vi "Helium Test - Step 4.vi"(7 "Step":i32, 8 "error in":errorcluster, 9 "Test Results":T9, 10 "Oil In":T1, 11 "Test Configuration":T2) -> (0 "error out":errorcluster, 1 "Test Results Out":T9, 2 "Oil Out":T1, 3 "Test Configuration Out":T2)   [LabVIEW 2015]
uses:
  Controls/Test Results.ctl
  Controls/Step Result.ctl
  Controls/Startup Test.ctl
  Controls/Test Information.ctl
  Controls/Vacuum Test.ctl
  Controls/Test Timing.ctl
  Controls/Vaccum Thresholds.ctl
  Controls/Helium Test.ctl
  Controls/Helium Thresholds.ctl
  Controls/Startup Thresholds.ctl
  CAN Communication/Oil/Typedefs/Session Handle.ctl
  CAN Communication/Oil/Oil.lvclass
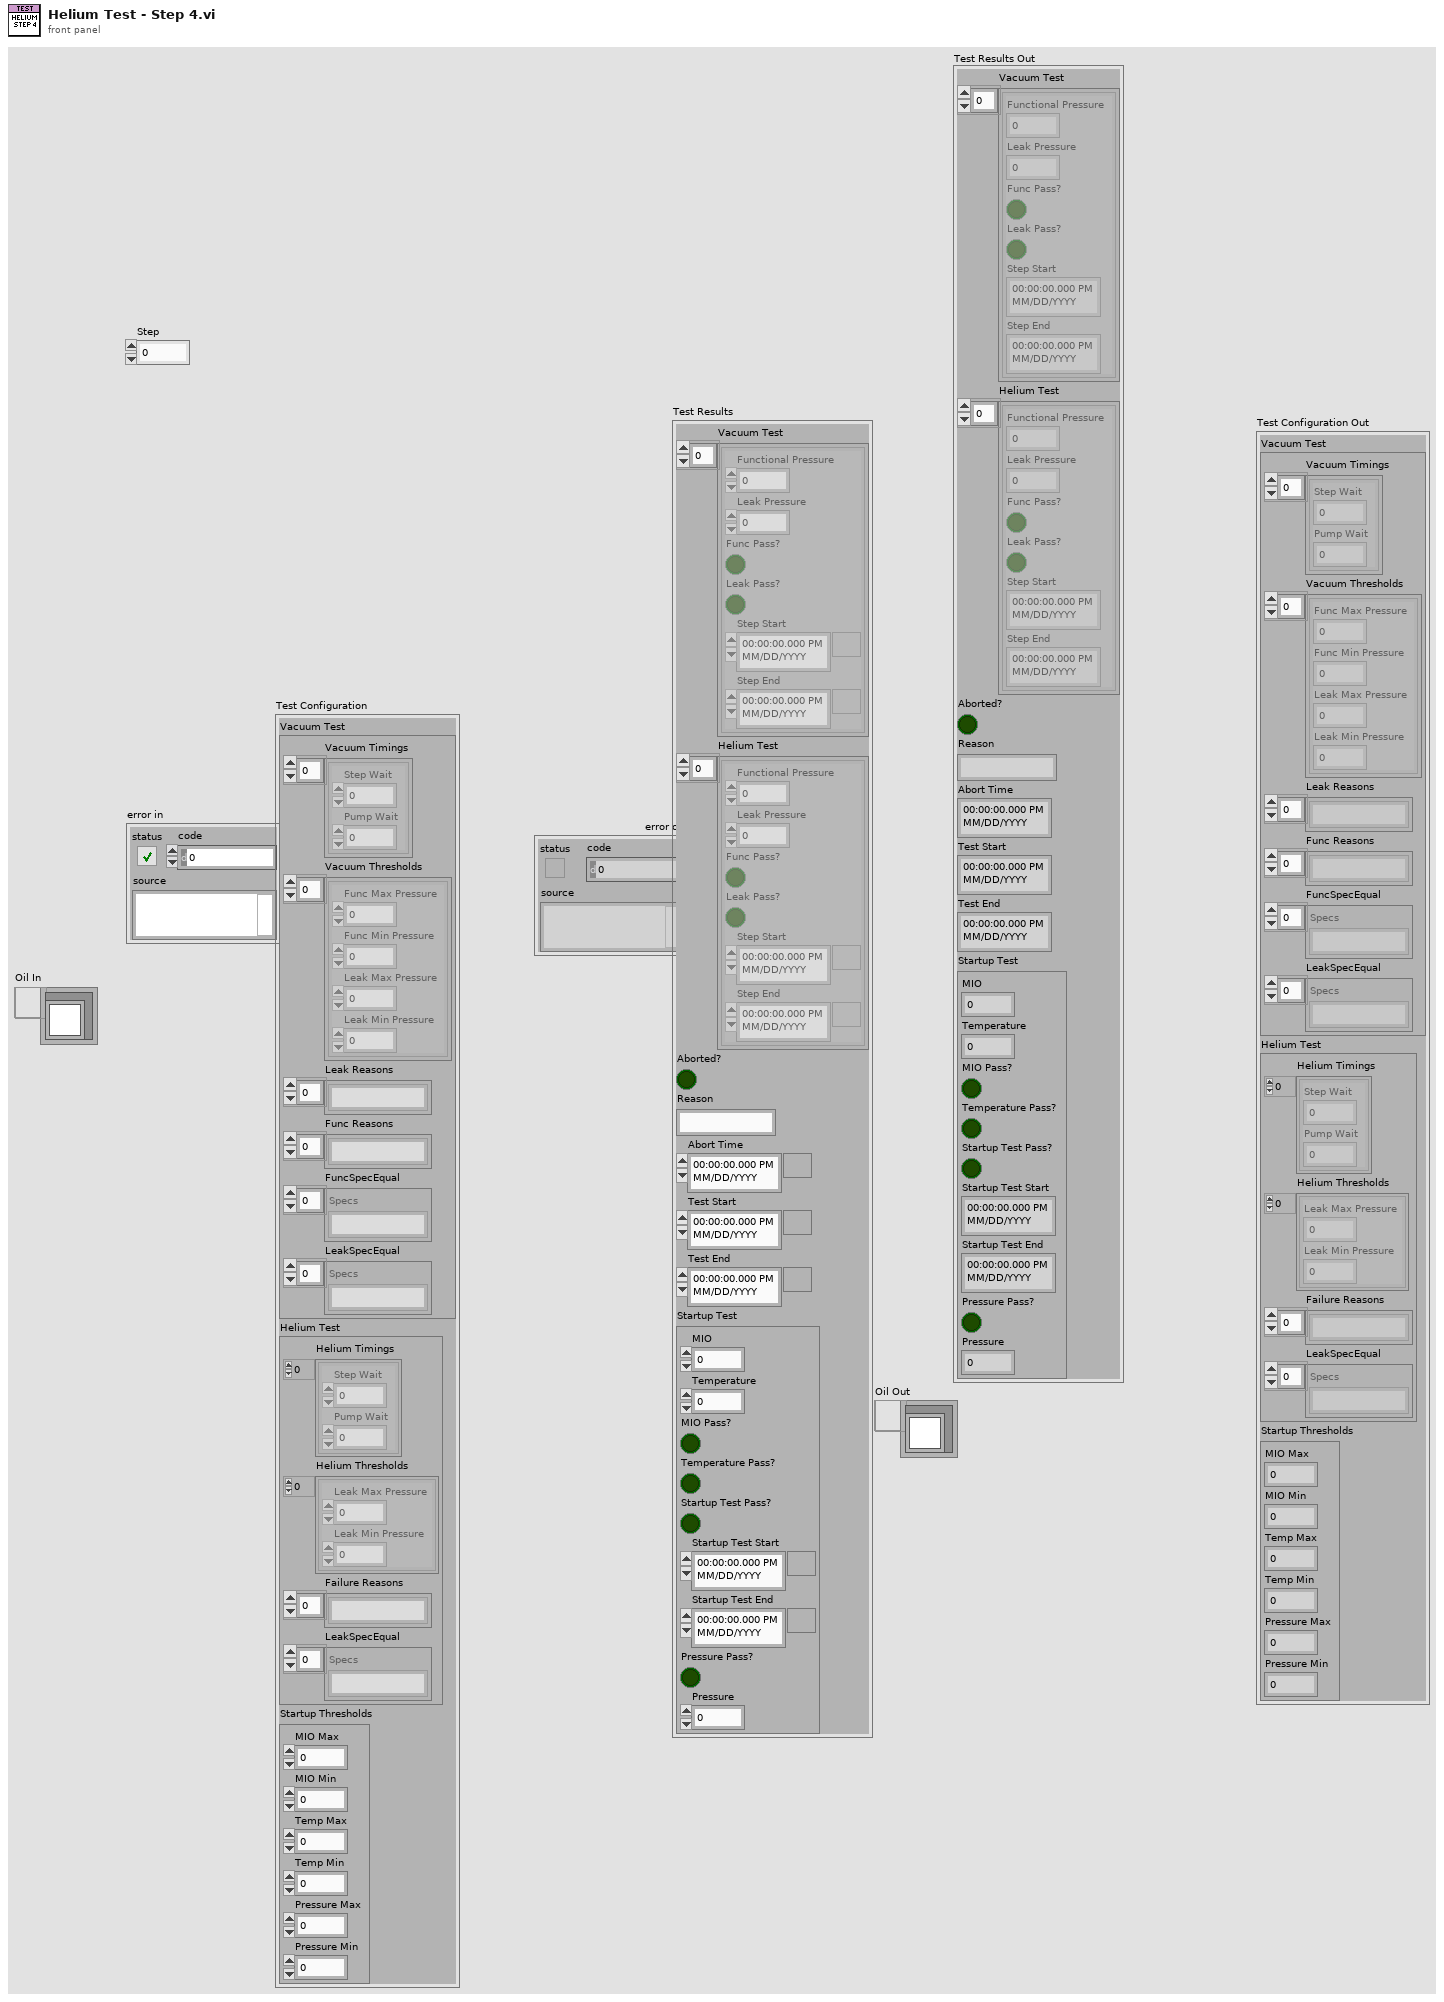
[diagram p1: front panel]
types:
  T1 = typedef "Oil.lvclass/Session Handle.ctl" = refnum<data-value>
  T2 = typedef "Test Information.ctl" = cluster{"Vacuum Test":T3, "Helium Test":T6, "Startup Thresholds":T8}
  T3 = typedef "Vacuum Test.ctl" = cluster{"Vacuum Timings":T4[], "Vacuum Thresholds":T5[], "Leak Reasons":string[], "Func Reasons":string[], "FuncSpecEqual":string[], "LeakSpecEqual":string[]}
  T4 = typedef "Test Timing.ctl" = cluster{"Step Wait":dbl, "Pump Wait":dbl}
  T5 = typedef "Vaccum Thresholds.ctl" = cluster{"Func Max Pressure":dbl, "Func Min Pressure":dbl, "Leak Max Pressure":dbl, "Leak Min Pressure":dbl}
  T6 = typedef "Helium Test.ctl" = cluster{"Helium Timings":T4[], "Helium Thresholds":T7[], "Failure Reasons":string[], "LeakSpecEqual":string[]}
  T7 = typedef "Helium Thresholds.ctl" = cluster{"Leak Max Pressure":dbl, "Leak Min Pressure":dbl}
  T8 = typedef "Startup Thresholds.ctl" = cluster{"MIO Max":dbl, "MIO Min":dbl, "Temp Max":dbl, "Temp Min":dbl, "Pressure Max":dbl, "Pressure Min":dbl}
  T9 = typedef "Test Results.ctl" = cluster{"Vacuum Test":T10[], "Helium Test":T10[], "Aborted?":bool, "Reason":string, "Abort Time":timestamp, "Test Start":timestamp, "Test End":timestamp, "Startup Test":T11}
  T10 = typedef "Step Result.ctl" = cluster{"Functional Pressure":dbl, "Leak Pressure":dbl, "Func Pass?":bool, "Leak Pass?":bool, "Step Start":timestamp, "Step End":timestamp}
  T11 = typedef "Startup Test.ctl" = cluster{"MIO":dbl, "Temperature":dbl, "MIO Pass?":bool, "Temperature Pass?":bool, "Startup Test Pass?":bool, "Startup Test Start":timestamp, "Startup Test End":timestamp, "Pressure Pass?":bool, "Pressure":dbl}
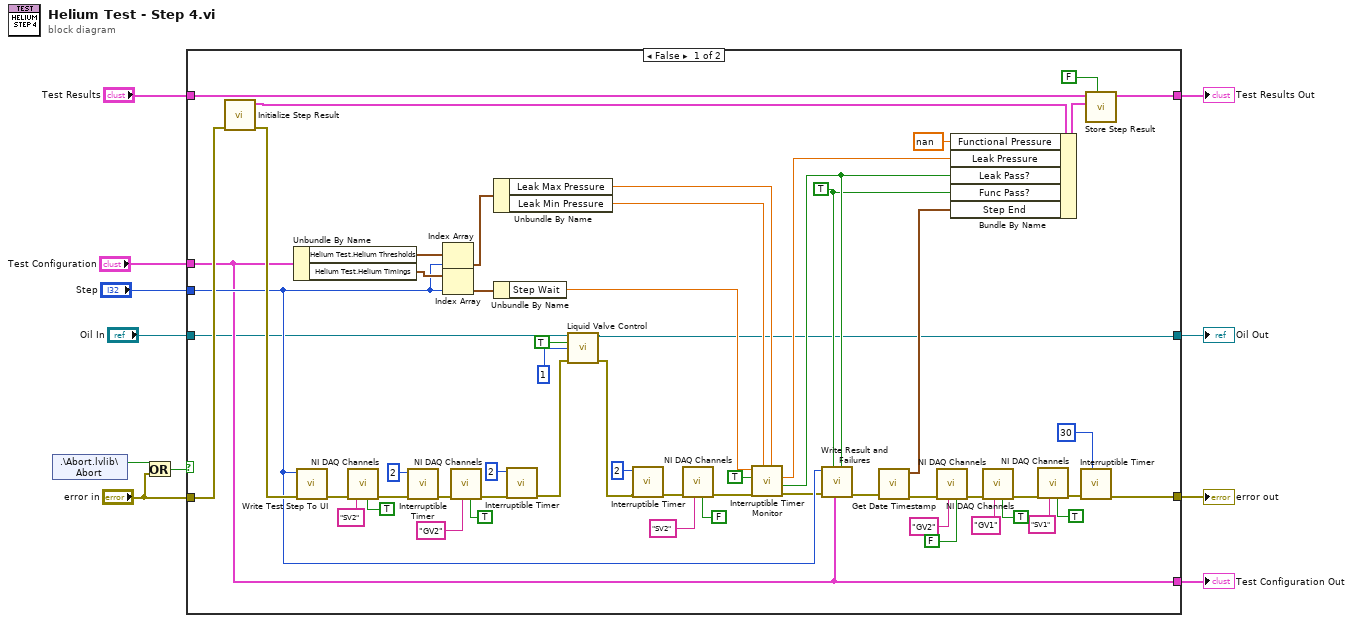
[diagram p0: block diagram]
diagram:
  n1 = shared-variable ".\\Abort.lvlib\\Abort"() -> (w10:bool)  [unwired: 1 in, 1 out]
  n2 = Or(x=w10, y="error in") -> (x .or. y?=w9:bool)
  n3 = case shown="False" w9 {
    tunnel: "error in" -> [w68 w71]
    tunnel: "Test Results" -> [w65 w72]
    tunnel: [w66 w72] -> w8
    tunnel: [w13 w71] -> w7
    tunnel: "Test Configuration" -> [w41 w70]
    tunnel: "Step" -> [w56 _]
    tunnel: [w41 w70] -> w3
    tunnel: [w27 w69] -> w1
    tunnel: "Oil In" -> [w35 w69]
    frame False {
      w43 = TRUE ("Func Pass?")
      n4 = call "Initialize Step Result.vi"("error in (no error)"=w68) -> ("error out"=w67:errorcluster, "New Step Result"=w64:T10)  [unwired: 8 in, 1 out]
      n5 = Unbundle By Name(w41) -> ("Helium Test.Helium Thresholds"=w61:T7[], "Helium Test.Helium Timings"=w60:T4[])
      n6 = call "Write Test Step To UI.vi"("error in (no error)"=w67, "Step"=w56) -> ("error out"=w54:errorcluster)  [unwired: 9 in]
      n7 = call "NI DAQ Channels.vi"("Control"=TRUE ("State"), "Channel"="SV2", "error in (no error)"=w54) -> ("error out"=w53:errorcluster)  [unwired: 7 in, 1 out]
      n8 = call "Interruptible Timer.vi"("error in (no error)"=w53, "Wait (s)"=2) -> ("error out"=w40:errorcluster)  [unwired: 7 in, 2 out]
      n9 = Index Array(array=w61, index=w56) -> (element=w57:T7)
      n10 = Index Array(array=w60, index=w56) -> (element=w59:T4)
      n11 = call "NI DAQ Channels.vi"("Control"=TRUE ("State"), "Channel"="GV2", "error in (no error)"=w40) -> ("error out"=w38:errorcluster)  [unwired: 7 in, 1 out]
      n12 = Unbundle By Name(w57) -> ("Leak Max Pressure"=w48:dbl, "Leak Min Pressure"=w49:dbl)
      n13 = Unbundle By Name(w59) -> ("Step Wait"=w51:dbl)
      n14 = call "Interruptible Timer.vi"("error in (no error)"=w38, "Wait (s)"=2) -> ("error out"=w34:errorcluster)  [unwired: 7 in, 2 out]
      n15 = call "Liquid Valve Control.vi"("Session Handle in"=w35, "On?"=TRUE, "Valve"=1, "error in (no error)"=w34) -> ("Session Handle out"=w27:T1, "error out"=w31:errorcluster)  [unwired: 8 in, 2 out]
      n16 = call "Interruptible Timer.vi"("error in (no error)"=w31, "Wait (s)"=2) -> ("error out"=w30:errorcluster)  [unwired: 7 in, 2 out]
      n17 = call "NI DAQ Channels.vi"("Control"=FALSE ("State"), "Channel"="SV2", "error in (no error)"=w30) -> ("error out"=w29:errorcluster)  [unwired: 7 in, 1 out]
      n18 = call "Interruptible Timer Monitor.vi"("Max"=w48, "Min"=w49, "error in (no error)"=w29, "Update UI?"=TRUE, "Wait (s)"=w51) -> ("error out"=w45:errorcluster, "In Range?"=w46:bool, "Leak Rate"=w47:dbl)  [unwired: 2 in, 2 out]
      n19 = call "Write Result and Failures.vi"("Leak"=w46, "Test Configuration"=w41, "Func"=w43, "error in (no error)"=w45, "Step"=w56) -> ("error out"=w28:errorcluster)  [unwired: 6 in]
      n20 = call "Get Date Timestamp.vi"("error in (no error)"=w28) -> ("error out"=w23:errorcluster, "current time"=w62:timestamp)  [unwired: 9 in]
      n21 = call "NI DAQ Channels.vi"("Control"=FALSE, "Channel"="GV2", "error in (no error)"=w23) -> ("error out"=w20:errorcluster)  [unwired: 7 in, 1 out]
      n22 = Bundle By Name(cluster=w64, "Functional Pressure"=nan, "Leak Pressure"=w47, "Leak Pass?"=w46, "Func Pass?"=w43, "Step End"=w62) -> (w63:T10)
      n23 = call "NI DAQ Channels.vi"("Control"=TRUE, "Channel"="GV1", "error in (no error)"=w20) -> ("error out"=w15:errorcluster)  [unwired: 7 in, 1 out]
      n24 = call "NI DAQ Channels.vi"("Control"=TRUE, "Channel"="SV1", "error in (no error)"=w15) -> ("error out"=w14:errorcluster)  [unwired: 7 in, 1 out]
      n25 = call "Interruptible Timer.vi"("error in (no error)"=w14, "Wait (s)"=30) -> ("error out"=w13:errorcluster)  [unwired: 7 in, 2 out]
      n26 = call "Store Step Result.vi"("Vacuum?"=FALSE, "Step Result"=w63, "Test Results In"=w65) -> ("Test Results Out"=w66:T9)  [unwired: 8 in]
    }
    frame True {
    }
  }
  "error out" <- w7
  "Test Results Out" <- w8
  "Test Configuration Out" <- w3
  "Oil Out" <- w1
